vi "Create.vi"(8 "error in (no error)":errorcluster) -> (0 "error out":errorcluster, 3 "Alarm DVR":refnum<data-value>)   [LabVIEW 2018, in "Alarm.lvclass"]
uses:
  Alarm.lvclass
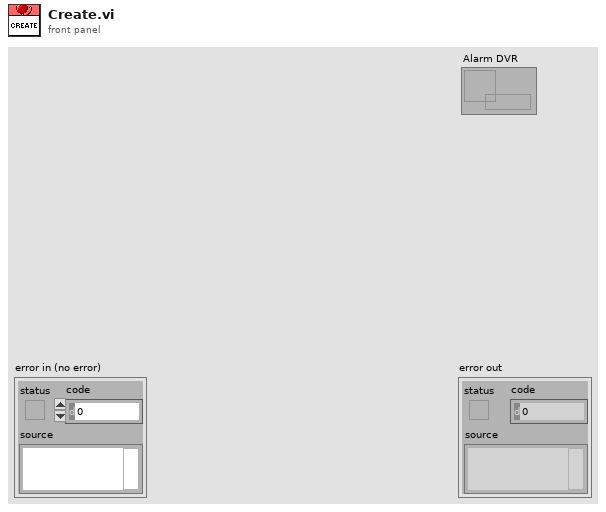
[diagram p1: front panel]
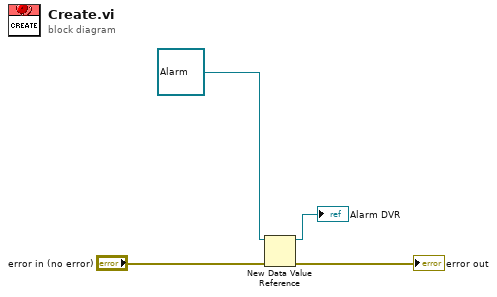
[diagram p0: block diagram]
diagram:
  n1 = New Data Value Reference(data value=refnum<class "Alarm.lvclass"> refnum ("Alarm in"), error in="error in (no error)") -> (data value reference=→"Alarm DVR":refnum<data-value>, error out=→"error out":errorcluster)
